vi "Analysis-SD.vi"() -> ()   [LabVIEW 2014]
uses:
  <vilib>/Utility/file.llb/Read From Spreadsheet File (DBL).vi
panel:
  out "média erro % 3":dbl=0.813672 format="%0.6f"
  out "média SD 3":dbl=0.022598000000000004 format="%0.6f"
  out "variance 3":dbl=1.1173453061224452e-05 format="%0.6f"
  out "standard deviation 3":dbl=0.00334267154551931 format="%0.6f"
  out "mean 3":dbl=2.7773959999999995 format="%0.4f"
  in  "file path (dialog if empty) 3":path=path "C:/users-lab/Andre/GITs/andretec/Z-Scan/medidas/z-teste-error-novos-5.txt"
  out "XY Graph 3":T1(graph)={"X Values"=[2.7709833333333336, 2.7733499999999998, 2.775716666666667, 2.778083333333333, 2.78045, 2.7828166666666663], "Histogram: h(x)"=[2, 9, 8, 16, 10, 5]}
  out "média erro % 2":dbl=0.75467 format="%0.6f"
  out "média SD 2":dbl=0.020952000000000002 format="%0.6f"
  out "variance 2":dbl=2.2137616326530615e-05 format="%0.6f"
  out "standard deviation 2":dbl=0.004705062839806777 format="%0.6f"
  out "mean 2":dbl=2.7757559999999994 format="%0.4f"
  in  "file path (dialog if empty) 2":path=path "C:/users-lab/Andre/GITs/andretec/Z-Scan/medidas/z-teste-error-novos-3.txt"
  out "XY Graph 2":T1(graph)={"X Values"=[2.7686083333333333, 2.7716250000000002, 2.7746416666666667, 2.7776583333333336, 2.780675, 2.783691666666667], "Histogram: h(x)"=[4, 13, 10, 10, 7, 6]}
  out "média erro %":dbl=0.7103659999999999 format="%0.6f"
  out "média SD":dbl=0.019738 format="%0.6f"
  out "variance":dbl=4.432490204081668e-05 format="%0.6f"
  out "standard deviation":dbl=0.006657694949516437 format="%0.6f"
  out "mean":dbl=2.778014 format="%0.4f"
  in  "file path (dialog if empty)":path=path "C:/users-lab/Andre/GITs/andretec/Z-Scan/medidas/z-teste-error-novos-1.txt"
  out "XY Graph":T1(graph)={"X Values"=[2.7660916666666666, 2.7718749999999996, 2.777658333333333, 2.7834416666666666, 2.7892249999999996, 2.795008333333333], "Histogram: h(x)"=[2, 15, 16, 11, 5, 1]}
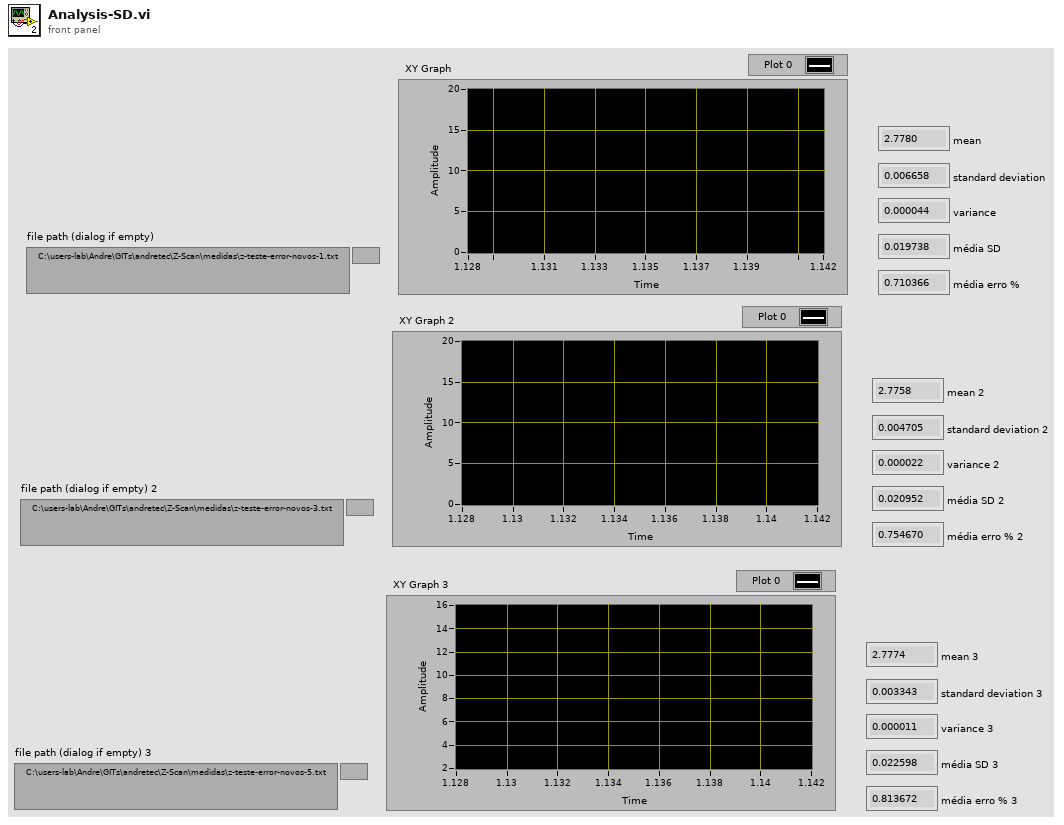
[diagram p1: front panel]
types:
  T1 = cluster{"X Values":dbl[], "Histogram: h(x)":i32[]}
  T2 = typedef "LVRangeTypeDef.ctl" = cluster{"Minimum":dbl, "Maximum":dbl, "Increment":dbl, "Minor Increment":dbl, "Start":dbl}
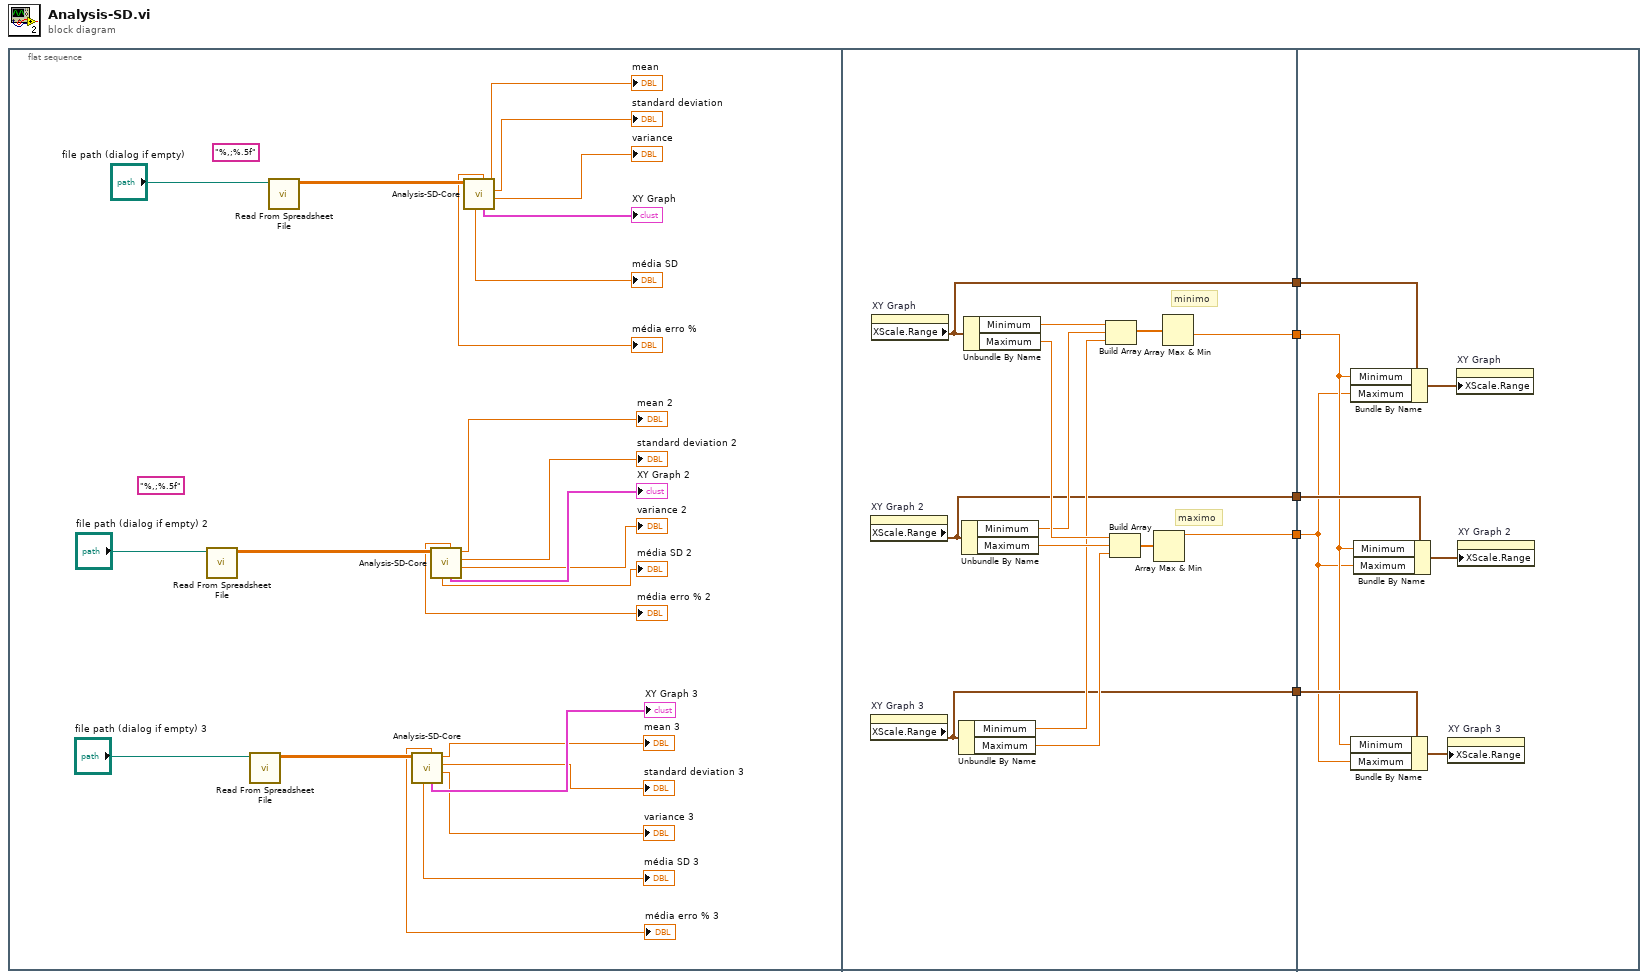
[diagram p0: block diagram]
diagram:
  n1 = flat-sequence {
    tunnel: [w34] -> w5
    tunnel: [w33] -> w4
    tunnel: [w32] -> w3
    tunnel: [w31] -> w2
    tunnel: [w30] -> w1
    tunnel: w5 -> [w44]
    tunnel: w4 -> [w49]
    tunnel: w3 -> [w48]
    tunnel: w2 -> [w43]
    tunnel: w1 -> [w46]
    frame #0 {
      (unwired) "%,;%.5f" ("format (%.3f)")
      (unwired) "%,;%.5f" ("format (%.3f)")
      n2 = call-poly <vilib>:"Read From Spreadsheet File.vi"("file path (dialog if empty)"="file path (dialog if empty) 2") -> ("all rows"=w20:dbl[][])  [unwired: 6 in, 4 out]
      n3 = call-poly <vilib>:"Read From Spreadsheet File.vi"("file path (dialog if empty)"="file path (dialog if empty) 3") -> ("all rows"=w12:dbl[][])  [unwired: 6 in, 4 out]
      n4 = call-poly <vilib>:"Read From Spreadsheet File.vi"("file path (dialog if empty)"="file path (dialog if empty)") -> ("all rows"=w29:dbl[][])  [unwired: 6 in, 4 out]
      n5 = call "Analysis-SD-Core.vi"("all rows"=w12) -> ("variance"=→"variance 3":dbl, "standard deviation"=→"standard deviation 3":dbl, "mean"=→"mean 3":dbl, "XY Graph"=→"XY Graph 3":T1, "média erro %"=→"média erro % 3":dbl, "média SD"=→"média SD 3":dbl)  [unwired: 5 in]
      n6 = call "Analysis-SD-Core.vi"("all rows"=w20) -> ("variance"=→"variance 2":dbl, "standard deviation"=→"standard deviation 2":dbl, "mean"=→"mean 2":dbl, "XY Graph"=→"XY Graph 2":T1, "média erro %"=→"média erro % 2":dbl, "média SD"=→"média SD 2":dbl)  [unwired: 5 in]
      n7 = call "Analysis-SD-Core.vi"("all rows"=w29) -> ("variance"=→"variance":dbl, "standard deviation"=→"standard deviation":dbl, "mean"=→"mean":dbl, "XY Graph"=→"XY Graph":T1, "média erro %"=→"média erro %":dbl, "média SD"=→"média SD":dbl)  [unwired: 5 in]
    }
    frame #1 {
      # "maximo"
      # "minimo"
      n8 = property on="XY Graph 2" class="XYGraph (strict)"() -> ("XScale.Range"=w32:T2)  [unwired: 2 in, 2 out]
      n9 = property on="XY Graph 3" class="XYGraph (strict)"() -> ("XScale.Range"=w30:T2)  [unwired: 2 in, 2 out]
      n10 = property on="XY Graph" class="XYGraph (strict)"() -> ("XScale.Range"=w33:T2)  [unwired: 2 in, 2 out]
      n11 = Unbundle By Name(w30) -> ("Minimum"=w37:dbl, "Maximum"=w41:dbl)
      n12 = Unbundle By Name(w32) -> ("Minimum"=w36:dbl, "Maximum"=w40:dbl)
      n13 = Unbundle By Name(w33) -> ("Minimum"=w35:dbl, "Maximum"=w39:dbl)
      n14 = Build Array(w35, w36, w37) -> (w38:dbl[])
      n15 = Build Array(w39, w40, w41) -> (w42:dbl[])
      n16 = Array Max & Min(array=w42) -> (max value=w31:dbl)  [unwired: 3 out]
      n17 = Array Max & Min(array=w38) -> (min value=w34:dbl)  [unwired: 3 out]
    }
    frame #2 {
      n18 = Bundle By Name(cluster=w49, "Minimum"=w44, "Maximum"=w43) -> (w50:T2)
      n19 = Bundle By Name(cluster=w46, "Minimum"=w44, "Maximum"=w43) -> (w45:T2)
      n20 = Bundle By Name(cluster=w48, "Minimum"=w44, "Maximum"=w43) -> (w47:T2)
      n21 = property on="XY Graph 3" class="XYGraph (strict)"("XScale.Range"=w45) -> ()  [unwired: 2 in, 2 out]
      n22 = property on="XY Graph" class="XYGraph (strict)"("XScale.Range"=w50) -> ()  [unwired: 2 in, 2 out]
      n23 = property on="XY Graph 2" class="XYGraph (strict)"("XScale.Range"=w47) -> ()  [unwired: 2 in, 2 out]
    }
  }
